vi "Start Purge Cycle.vi"(8 "error in (no error)":errorcluster, 10 "Period (500)":i32=500 min=1 max=999, 11 "VISA resource name":refnum<visa-resource-name>) -> (0 "error out":errorcluster, 3 "VISA resource name out":refnum<visa-resource-name>)   [LabVIEW 2023, in "Fluke Molbox 1 Plus.lvlib"]
doc: "Start a purge cycle. THe purge cycle takes the specified time period to complete. The cycle must be completed or aborted using the Abort VI before performing another operation."
uses:
  Fluke Molbox 1 Plus.lvlib
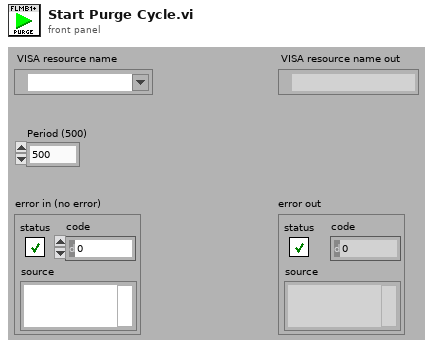
[diagram p1: front panel]
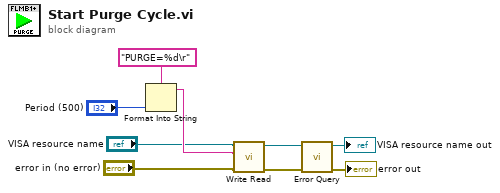
[diagram p0: block diagram]
diagram:
  n1 = Format Into String(format string="PURGE=%d\r", "Period (500)") -> (resulting string=w2:string)  [unwired: 2 in, 1 out]
  n2 = call "Write Read.vi"("error in (no error)"="error in (no error)", "Write String"=w2, "VISA resource name"="VISA resource name") -> ("error out"=w4:errorcluster, "VISA resource name out"=w5:refnum<visa-resource-name>)  [unwired: 6 in, 1 out]
  n3 = call "Error Query.vi"("error in (no error)"=w4, "VISA resource name"=w5) -> ("error out"=→"error out":errorcluster, "VISA resource name out"=→"VISA resource name out":refnum<visa-resource-name>)  [unwired: 6 in, 2 out]
